vi "功能试验 数据分离.vi"(10 "扭矩":dbl[](array[numeric]), 11 "角度":dbl[](array[numeric])) -> (1 "扭矩右转2":dbl[](array[numeric]), 2 "扭矩左转":dbl[](array[numeric]), 3 "扭矩右转1":dbl[](array[numeric]))   [LabVIEW 2015, in "Logging.lvlib"]
uses:
  Logging.lvlib
  <vilib>/Analysis/1siggen.llb/Ramp Pattern by Samples.vi
  <vilib>/Analysis/NI_AALBase.lvlib
  <vilib>/gmath/NI_Gmath.lvlib
panel:
  in  "细分因子":dbl=1.0
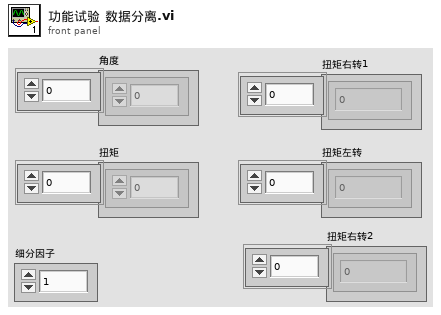
[diagram p1: front panel]
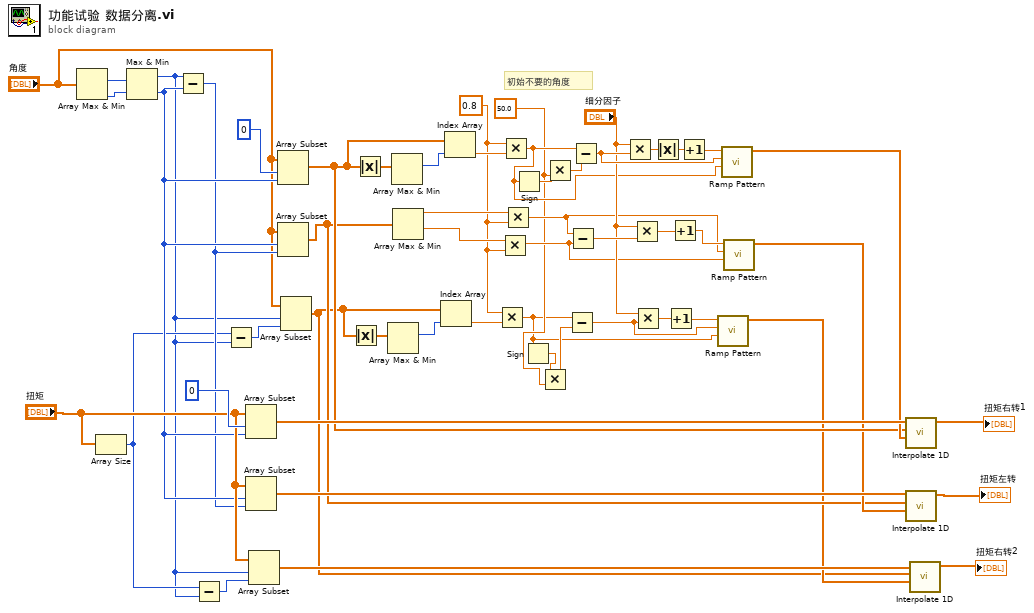
[diagram p0: block diagram]
diagram:
  w8 = 50.0 ("y")
  w28 = 0.8 ("x")
  # "初始不要的角度"
  n1 = Array Max & Min(array="角度") -> (max index (indices)=w53:i32, min index (indices)=w52:i32)  [unwired: 2 out]
  n2 = Array Size(array="扭矩") -> (size(s)=w44:i32)
  n3 = Max & Min(x=w53, y=w52) -> (max(x,y)=w43:i32, min(x,y)=w46:i32)
  n4 = Subtract(x=w43, y=w46) -> (x-y=w45:i32)
  n5 = Subtract(x=w44, y=w43) -> (x-y=w50:i32)
  n6 = Subtract(x=w44, y=w43) -> (x-y=w47:i32)
  n7 = Array Subset(array="扭矩", index=0 ("索引"), length=w46) -> (w21:dbl[])
  n8 = Array Subset(array="扭矩", index=w46, length=w45) -> (w5:dbl[])
  n9 = Array Subset(array="扭矩", index=w43, length=w50) -> (w18:dbl[])
  n10 = Array Subset(array="角度", index=0 ("索引"), length=w46) -> (w15:dbl[])
  n11 = Array Subset(array="角度", index=w46, length=w45) -> (w3:dbl[])
  n12 = Array Subset(array="角度", index=w43, length=w47) -> (w1:dbl[])
  n13 = Absolute Value(x=w1) -> (abs(x)=w36:dbl[])
  n14 = Absolute Value(x=w15) -> (abs(x)=w41:dbl[])
  n15 = Array Max & Min(array=w36) -> (max index (indices)=w35:i32)  [unwired: 3 out]
  n16 = Array Max & Min(array=w41) -> (max index (indices)=w40:i32)  [unwired: 3 out]
  n17 = Array Max & Min(array=w3) -> (max value=w30:dbl, min value=w29:dbl)  [unwired: 2 out]
  n18 = Index Array(array=w1, index=w35) -> (element=w34:dbl)
  n19 = Index Array(array=w15, index=w40) -> (element=w39:dbl)
  n20 = Multiply(x=w28, y=w34) -> (x*y=w6:dbl)
  n21 = Multiply(x=w29, y=w28) -> (x*y=w22:dbl)
  n22 = Multiply(x=w28, y=w39) -> (x*y=w10:dbl)
  n23 = Multiply(x=w30, y=w28) -> (x*y=w23:dbl)
  n24 = Sign(1:w10) -> (0:w12:dbl)
  n25 = Sign(1:w6) -> (0:w9:dbl)
  n26 = Multiply(x=w9, y=w8) -> (x*y=w7:dbl)
  n27 = Multiply(x=w12, y=w8) -> (x*y=w11:dbl)
  n28 = Subtract(x=w6, y=w7) -> (x-y=w31:dbl)
  n29 = Subtract(x=w23, y=w22) -> (x-y=w27:dbl)
  n30 = Subtract(x=w10, y=w11) -> (x-y=w37:dbl)
  n31 = Multiply(x="细分因子", y=w37) -> (x*y=w14:dbl)
  n32 = Multiply(x="细分因子", y=w27) -> (x*y=w25:dbl)
  n33 = Multiply(x="细分因子", y=w31) -> (x*y=w33:dbl)
  n34 = Absolute Value(x=w14) -> (abs(x)=w13:dbl)
  n35 = Increment(x=w33) -> (x+1=w32:dbl)
  n36 = Increment(x=w25) -> (x+1=w24:dbl)
  n37 = Increment(x=w13) -> (x+1=w38:dbl)
  n38 = call-poly <vilib>:"Ramp Pattern.vi"("start"=w6, "end"=w31, "samples"=w32) -> ("Ramp Pattern"=w2:dbl[])  [unwired: 7 in, 1 out]
  n39 = call-poly <vilib>:"Ramp Pattern.vi"("start"=w10, "end"=w37, "samples"=w38) -> ("Ramp Pattern"=w16:dbl[])  [unwired: 7 in, 1 out]
  n40 = call-poly <vilib>:"Ramp Pattern.vi"("start"=w22, "end"=w23, "samples"=w24) -> ("Ramp Pattern"=w4:dbl[])  [unwired: 7 in, 1 out]
  n41 = call <vilib>:"Interpolate 1D.vi"("xi"=w16, "X"=w15, "Y"=w21) -> ("yi"=→"扭矩右转1":dbl[])  [unwired: 6 in, 2 out]
  n42 = call <vilib>:"Interpolate 1D.vi"("xi"=w4, "X"=w3, "Y"=w5) -> ("yi"=→"扭矩左转":dbl[])  [unwired: 6 in, 2 out]
  n43 = call <vilib>:"Interpolate 1D.vi"("xi"=w2, "X"=w1, "Y"=w18) -> ("yi"=→"扭矩右转2":dbl[])  [unwired: 6 in, 2 out]
